vi "Create RPC Method.vi"(8 "error in (no error)":errorcluster, 10 "RPC Method Parameters":T1, 11 "Server class in":refnum<vi>) -> (0 "error out":errorcluster, 2 "Newly created ?":bool, 3 "Server class out":refnum<vi>)   [LabVIEW 2019, in "gRPC Scripting Tools.lvlib"]
uses:
  gRPC Scripting Tools.lvlib
  TypeDefs/RPC Method Parameters.ctl
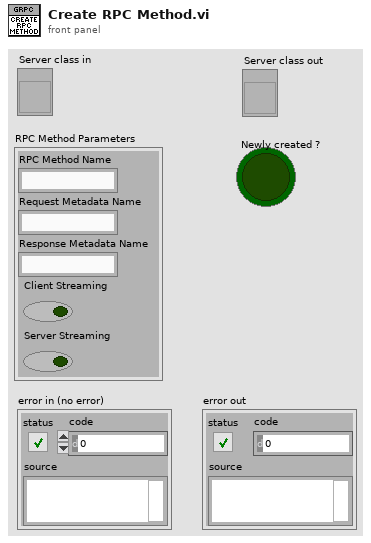
[diagram p1: front panel]
types:
  T1 = typedef "gRPC Scripting Tools.lvlib/RPC Method Parameters.ctl" = cluster{"RPC Method Name":string, "Request Metadata Name":string, "Response Metadata Name":string, "Client Streaming":bool, "Server Streaming":bool}
  T2 = enum32{"invalid VI type", "Standard VI", "Control VI", "Global VI", "Polymorphic VI", "Configuration VI", "SubSystem", "Facade VI", "Method VI"}
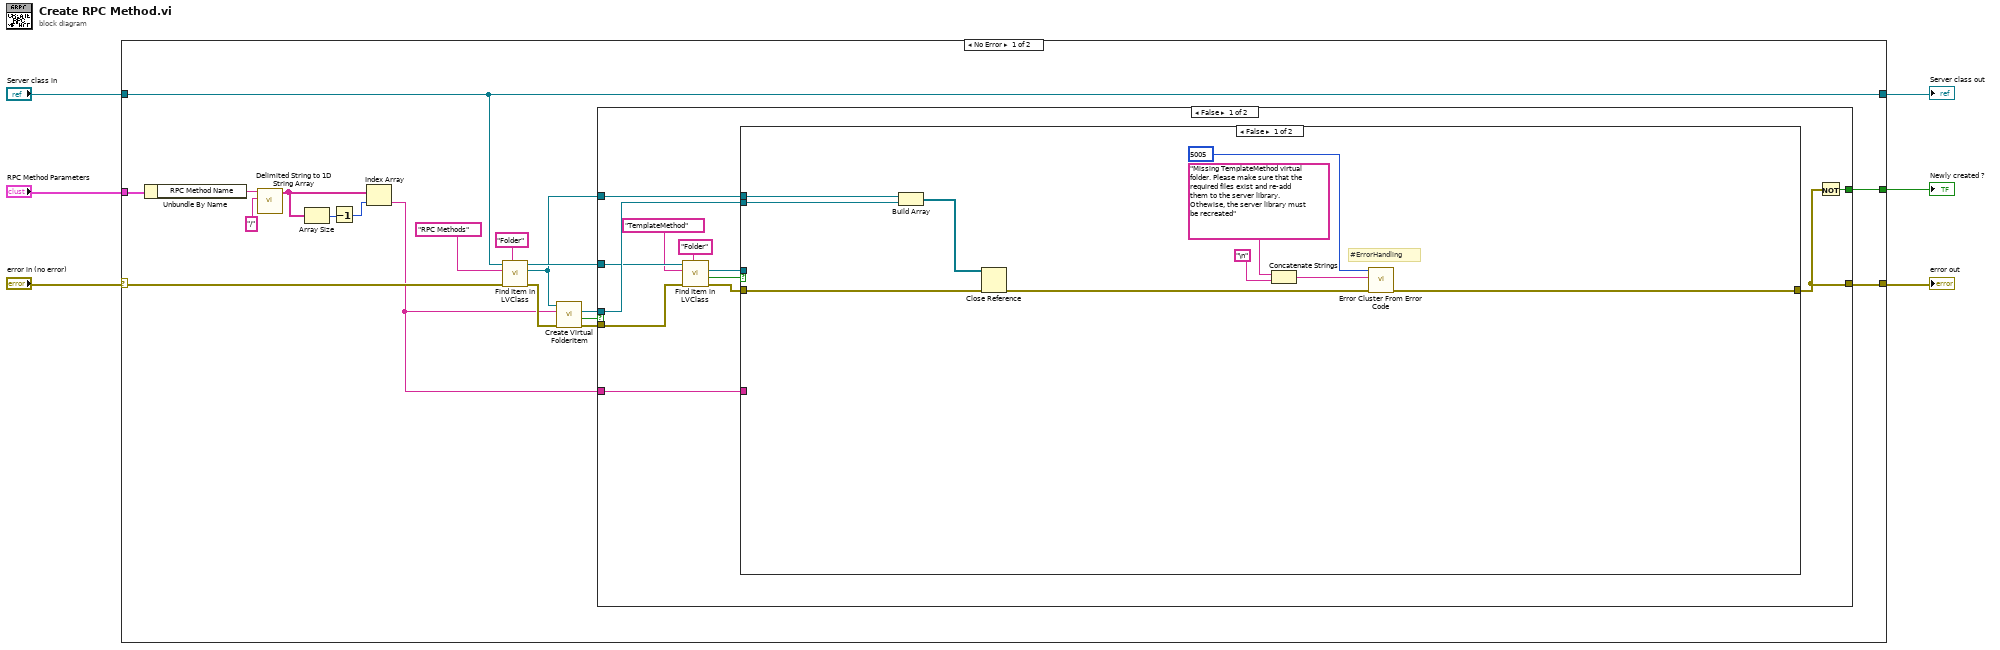
[diagram p0: block diagram]
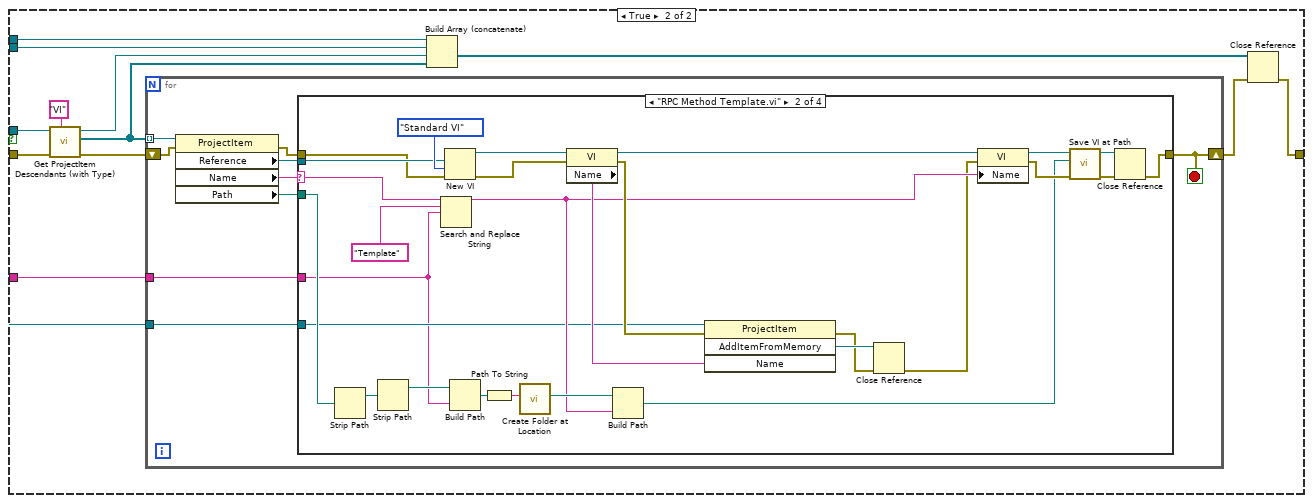
[diagram p2: hidden frame]
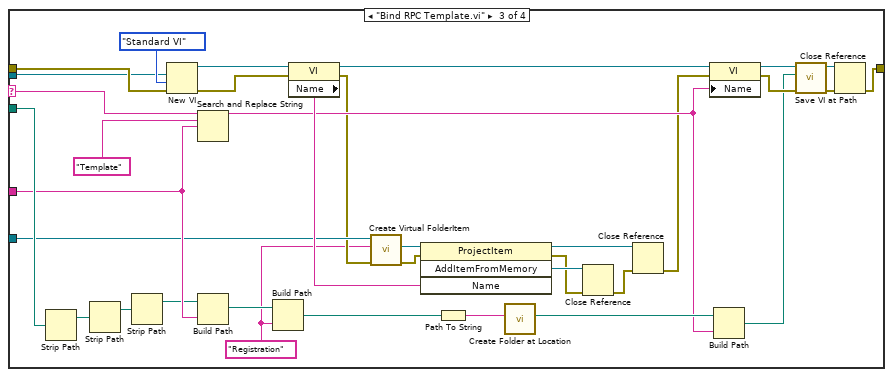
[diagram p4: hidden frame]
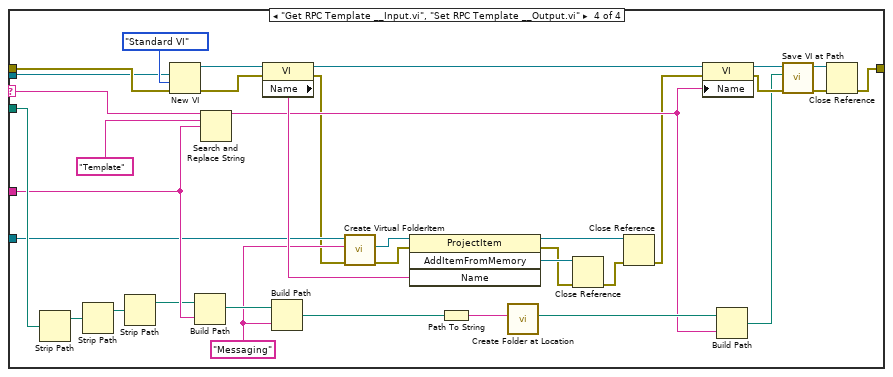
[diagram p5: hidden frame]
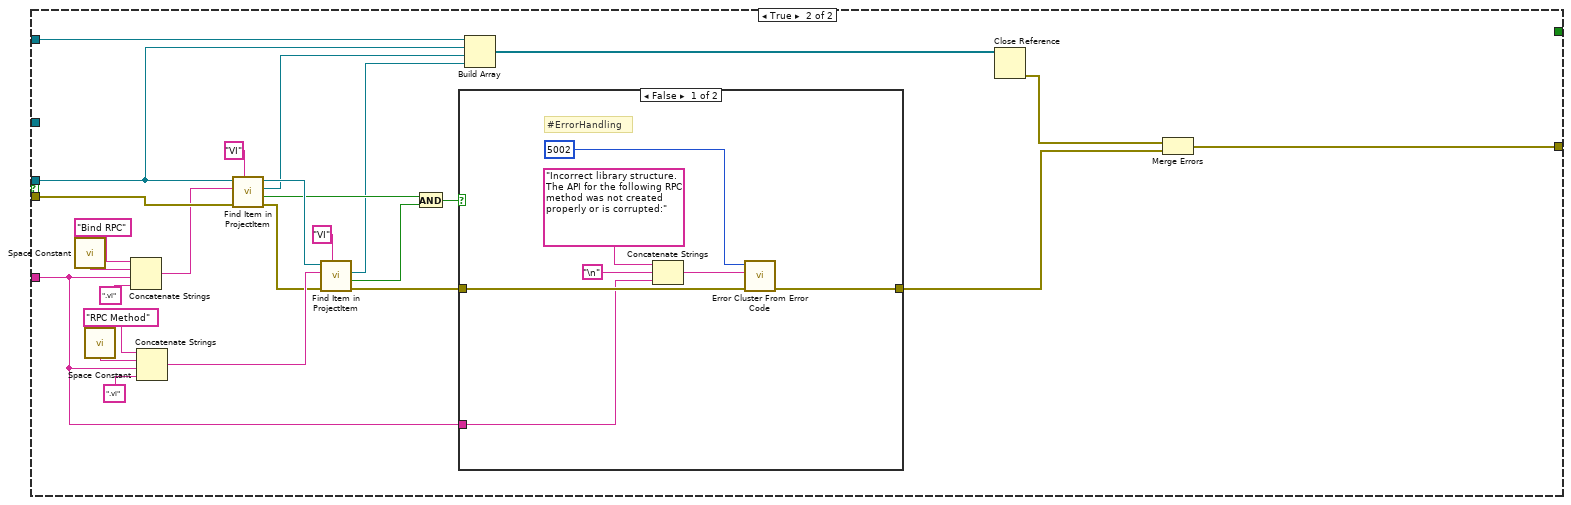
[diagram p6: hidden frame]
diagram:
  n1 = case shown="No Error" "error in (no error)" {
    selector: "error in (no error)" -> [w16 w203]
    tunnel: "Server class in" -> [w15 w202]
    tunnel: [w21 w203] -> w5
    tunnel: [w15 w202] -> w3
    tunnel: [w14 _] -> w2
    tunnel: "RPC Method Parameters" -> [w7 _]
    frame No Error {
      n2 = Unbundle By Name(w7) -> ("RPC Method Name"=w10:string)
      n3 = call <vilib>:"Delimited String to 1D String Array.vi"("delimiter"="/", "delimited string"=w10) -> ("string array"=w13:string[])  [unwired: 9 in]
      n4 = Array Size(array=w13) -> (size(s)=w11:i32)
      n5 = Decrement(x=w11) -> (x-1=w12:i32)
      n6 = Index Array(array=w13, index=w12) -> (element=w8:string)
      n7 = call "Find Item in LVClass.vi"("Item Type"="Folder", "error in (no error)"=w16, "Item Name"="RPC Methods", "Class Item in"=w15) -> ("error out"=w20:errorcluster, "Project Item (Class Item)"=w18:refnum<vi>, "Class Item out"=w22:refnum<vi>)  [unwired: 4 in, 1 out]
      n8 = call "Create Virtual FolderItem.vi"("error in (no error)"=w20, "Folder Name"=w8, "ProjectItem in"=w18) -> ("error out"=w19:errorcluster, "Already exists?"=w25:bool, "FolderItem reference out"=w17:refnum<vi>)  [unwired: 5 in, 1 out]
      n9 = case shown="False" w25 {
        tunnel: w17 -> [w37 w176]
        tunnel: w18 -> [w36 w177]
        tunnel: w19 -> [w35 w192]
        tunnel: [w30 w168] -> w21
        tunnel: w22 -> [w34 _]
        tunnel: w8 -> [w31 w172]
        tunnel: [w29 _] -> w14
        frame False {
          n10 = call "Find Item in LVClass.vi"("Item Type"="Folder", "error in (no error)"=w35, "Item Name"="TemplateMethod", "Class Item in"=w34) -> ("error out"=w27:errorcluster, "Found?"=w26:bool, "Project Item (Class Item)"=w28:refnum<vi>)  [unwired: 4 in, 1 out]
          n11 = case shown="False" w26 {
            tunnel: w37 -> [w41 w59]
            tunnel: w36 -> [w42 w58]
            tunnel: w31 -> [_ w56]
            tunnel: [w43 w55] -> w30
            tunnel: w28 -> [_ w54]
            tunnel: w27 -> [w40 w53]
            frame False {
              # "#ErrorHandling"
              n12 = Build Array(w42, w41) -> (w39:refnum<vi>[])
              n13 = Close Reference(reference=w39, error in (no error)=w40) -> (error out=w38:errorcluster)
              n14 = Concatenate Strings("Missing TemplateMethod virtual folder. Please make sure that the required files exist and re-add them to the server library. Othewise, the server library must be recreated" ("error message (\"\")"), "\n") -> (w44:string)
              n15 = call <vilib>:"Error Cluster From Error Code.vi"("error in (no error)"=w38, "error message (\"\")"=w44, "error code (0)"=5005) -> ("error out"=w43:errorcluster)  [unwired: 6 in]
            }
            frame True {
              n16 = call "Get ProjectItem Descendants (with Type).vi"("Type"="VI", "error in (no error)"=w53, "ProjectItem in"=w54) -> ("error out"=w49:errorcluster, "All Descendents"=w50:refnum<vi>[], "ProjectItem out"=w51:refnum<vi>)  [unwired: 6 in]
              n17 = for {
                tunnel: w50 -> [w68] mode=indexing
                tunnel: w59 -> [w62]
                tunnel: w56 -> [w63]
                shift-right: [w60] -> w48
                shift-left: w49 -> [w67]
                stop <- w60 stop-if-true
                n18 = property class="ProjectItem"(reference=w68, error in=w67) -> (error out=w61:errorcluster, "Reference"=w65:refnum<vi>, "Name"=w66:string, "Path"=w64:path)  [unwired: 1 out]
                n19 = case shown="\"RPC Method Template.vi\"" w66 {
                  selector: w66 -> [_ w75 w113 w146]
                  tunnel: w65 -> [_ w76 w114 w147]
                  tunnel: w64 -> [_ w74 w112 w145]
                  tunnel: w63 -> [_ w70 w111 w144]
                  tunnel: w62 -> [_ w73 w105 w140]
                  tunnel: w61 -> [w69 w72 w115 w148]
                  tunnel: [w69 w71 w108 w143] -> w60
                  frame "None", Default {
                  }
                  frame "RPC Method Template.vi" {
                    n20 = Strip Path(path=w74) -> (stripped path=w77:path)  [unwired: 1 out]
                    n21 = Strip Path(path=w77) -> (stripped path=w88:path)  [unwired: 1 out]
                    n22 = Search and Replace String(input string=w75, search string="Template", replace string=w70) -> (result string=w84:string)  [unwired: 5 in, 3 out]
                    n23 = New VI(8:w72, 9:T2."Standard VI" ("vi type (standard vi)"), 10:w76) -> (0:w92:errorcluster, 3:w95:refnum<vi>)  [unwired: 1 in, 3 out]
                    n24 = Build Path(base path=w88, name or relative path=w70) -> (appended path=w87:path)
                    n25 = Path To String(path=w87) -> (string=w86:string)
                    n26 = call "Create Folder at Location.vi"("Path"=w86) -> ("Full path out"=w85:path)  [unwired: 8 in, 2 out]
                    n27 = property class="VI"(reference=w95, error in=w92) -> (reference out=w93:refnum<vi>, error out=w91:errorcluster, "Name"=w96:string)
                    n28 = Build Path(base path=w85, name or relative path=w84) -> (appended path=w83:path)
                    n29 = invoke class="ProjectItem" method="AddItemFromMemory"(reference=w73, error in=w91, "Name"=w96) -> (error out=w79:errorcluster, "AddItemFromMemory"=w80:refnum<vi>)  [unwired: 1 in, 2 out]
                    n30 = Close Reference(reference=w80, error in (no error)=w79) -> (error out=w78:errorcluster)
                    n31 = property class="VI"(reference=w93, error in=w78, "Name"=w84) -> (reference out=w90:refnum<vi>, error out=w89:errorcluster)
                    n32 = call "Save VI at Path.vi"("error in (no error)"=w89, "Path"=w83, "VI in"=w90) -> ("error out"=w82:errorcluster, "VI out"=w81:refnum<vi>)  [unwired: 6 in, 1 out]
                    n33 = Close Reference(reference=w81, error in (no error)=w82) -> (error out=w71:errorcluster)
                  }
                  frame "Bind RPC Template.vi" {
                    w103 = "Registration" ("name or relative path")
                    n34 = Strip Path(path=w112) -> (stripped path=w116:path)  [unwired: 1 out]
                    n35 = Strip Path(path=w116) -> (stripped path=w107:path)  [unwired: 1 out]
                    n36 = Strip Path(path=w107) -> (stripped path=w106:path)  [unwired: 1 out]
                    n37 = New VI(8:w115, 9:T2."Standard VI" ("vi type (standard vi)"), 10:w114) -> (0:w127:errorcluster, 3:w130:refnum<vi>)  [unwired: 1 in, 3 out]
                    n38 = Search and Replace String(input string=w113, search string="Template", replace string=w111) -> (result string=w122:string)  [unwired: 5 in, 3 out]
                    n39 = Build Path(base path=w106, name or relative path=w111) -> (appended path=w110:path)
                    n40 = Build Path(base path=w110, name or relative path=w103) -> (appended path=w109:path)
                    n41 = property class="VI"(reference=w130, error in=w127) -> (reference out=w128:refnum<vi>, error out=w104:errorcluster, "Name"=w131:string)
                    n42 = call "Create Virtual FolderItem.vi"("error in (no error)"=w104, "Folder Name"=w103, "ProjectItem in"=w105) -> ("error out"=w101:errorcluster, "FolderItem reference out"=w102:refnum<vi>)  [unwired: 5 in, 2 out]
                    n43 = invoke class="ProjectItem" method="AddItemFromMemory"(reference=w102, error in=w101, "Name"=w131) -> (reference out=w100:refnum<vi>, error out=w117:errorcluster, "AddItemFromMemory"=w118:refnum<vi>)  [unwired: 1 in, 1 out]
                    n44 = Path To String(path=w109) -> (string=w124:string)
                    n45 = call "Create Folder at Location.vi"("Path"=w124) -> ("Full path out"=w123:path)  [unwired: 8 in, 2 out]
                    n46 = Close Reference(reference=w118, error in (no error)=w117) -> (error out=w99:errorcluster)
                    n47 = Close Reference(reference=w100, error in (no error)=w99) -> (error out=w98:errorcluster)
                    n48 = property class="VI"(reference=w128, error in=w98, "Name"=w122) -> (reference out=w126:refnum<vi>, error out=w125:errorcluster)
                    n49 = Build Path(base path=w123, name or relative path=w122) -> (appended path=w121:path)
                    n50 = call "Save VI at Path.vi"("error in (no error)"=w125, "Path"=w121, "VI in"=w126) -> ("error out"=w120:errorcluster, "VI out"=w119:refnum<vi>)  [unwired: 6 in, 1 out]
                    n51 = Close Reference(reference=w119, error in (no error)=w120) -> (error out=w108:errorcluster)
                  }
                  frame "Get RPC Template __Input.vi", "Set RPC Template __Output.vi" {
                    w137 = "Messaging" ("name or relative path")
                    n52 = Strip Path(path=w145) -> (stripped path=w151:path)  [unwired: 1 out]
                    n53 = Strip Path(path=w151) -> (stripped path=w142:path)  [unwired: 1 out]
                    n54 = Strip Path(path=w142) -> (stripped path=w141:path)  [unwired: 1 out]
                    n55 = New VI(8:w148, 9:T2."Standard VI" ("vi type (standard vi)"), 10:w147) -> (0:w162:errorcluster, 3:w165:refnum<vi>)  [unwired: 1 in, 3 out]
                    n56 = Build Path(base path=w141, name or relative path=w144) -> (appended path=w150:path)
                    n57 = Search and Replace String(input string=w146, search string="Template", replace string=w144) -> (result string=w157:string)  [unwired: 5 in, 3 out]
                    n58 = property class="VI"(reference=w165, error in=w162) -> (reference out=w163:refnum<vi>, error out=w136:errorcluster, "Name"=w166:string)
                    n59 = Build Path(base path=w150, name or relative path=w137) -> (appended path=w149:path)
                    n60 = call "Create Virtual FolderItem.vi"("error in (no error)"=w136, "Folder Name"=w137, "ProjectItem in"=w140) -> ("error out"=w138:errorcluster, "FolderItem reference out"=w139:refnum<vi>)  [unwired: 5 in, 2 out]
                    n61 = invoke class="ProjectItem" method="AddItemFromMemory"(reference=w139, error in=w138, "Name"=w166) -> (reference out=w135:refnum<vi>, error out=w152:errorcluster, "AddItemFromMemory"=w153:refnum<vi>)  [unwired: 1 in, 1 out]
                    n62 = Path To String(path=w149) -> (string=w159:string)
                    n63 = call "Create Folder at Location.vi"("Path"=w159) -> ("Full path out"=w158:path)  [unwired: 8 in, 2 out]
                    n64 = Close Reference(reference=w153, error in (no error)=w152) -> (error out=w134:errorcluster)
                    n65 = Close Reference(reference=w135, error in (no error)=w134) -> (error out=w133:errorcluster)
                    n66 = property class="VI"(reference=w163, error in=w133, "Name"=w157) -> (reference out=w161:refnum<vi>, error out=w160:errorcluster)
                    n67 = Build Path(base path=w158, name or relative path=w157) -> (appended path=w156:path)
                    n68 = call "Save VI at Path.vi"("error in (no error)"=w160, "Path"=w156, "VI in"=w161) -> ("error out"=w155:errorcluster, "VI out"=w154:refnum<vi>)  [unwired: 6 in, 1 out]
                    n69 = Close Reference(reference=w154, error in (no error)=w155) -> (error out=w143:errorcluster)
                  }
                }
              }
              n70 = Build Array (concatenate)(w58, w59, w51, w50) -> (w57:refnum<vi>[])
              n71 = Close Reference(reference=w57, error in (no error)=w48) -> (error out=w55:errorcluster)
            }
          }
          n72 = Not(x=w30) -> (.not. x?=w29:bool)
        }
        frame True {
          n73 = call <vilib>:"Space Constant.vi"() -> ("String"=w185:string)
          n74 = call <vilib>:"Space Constant.vi"() -> ("String"=w184:string)
          n75 = Concatenate Strings("Bind RPC" ("string"), w185, w172, ".vi" ("string")) -> (w188:string)
          n76 = Concatenate Strings("RPC Method" ("string"), w184, w172, ".vi" ("string")) -> (w182:string)
          n77 = call "Find Item in ProjectItem.vi"("Item Type"="VI" ("Type"), "error in (no error)"=w192, "Name"=w188, "ProjectItem in"=w176) -> ("error out"=w181:errorcluster, "Found ?"=w180:bool, "Item Refnum out"=w175:refnum<vi>, "ProjectItem out"=w190:refnum<vi>)  [unwired: 4 in]
          n78 = call "Find Item in ProjectItem.vi"("Item Type"="VI" ("Type"), "error in (no error)"=w181, "Name"=w182, "ProjectItem in"=w190) -> ("error out"=w173:errorcluster, "Found ?"=w179:bool, "Item Refnum out"=w174:refnum<vi>)  [unwired: 4 in, 1 out]
          n79 = And(x=w180, y=w179) -> (x .and. y?=w178:bool)
          n80 = case shown="False" w178 {
            tunnel: w173 -> [w200 w201]
            tunnel: w172 -> [w196 _]
            tunnel: [w194 w201] -> w170
            frame False {
              # "#ErrorHandling"
              n81 = Concatenate Strings("Incorrect library structure. The API for the following RPC method was not created properly or is corrupted:" ("error message (\"\")"), "\n", w196) -> (w195:string)
              n82 = call <vilib>:"Error Cluster From Error Code.vi"("error in (no error)"=w200, "error message (\"\")"=w195, "error code (0)"=5002) -> ("error out"=w194:errorcluster)  [unwired: 6 in]
            }
            frame True {
            }
          }
          n83 = Build Array(w177, w176, w175, w174) -> (w171:refnum<vi>[])
          n84 = Close Reference(reference=w171) -> (error out=w169:errorcluster)  [unwired: 1 in]
          n85 = Merge Errors(w169, w170) -> (w168:errorcluster)
        }
      }
    }
    frame Error {
    }
  }
  "error out" <- w5
  "Server class out" <- w3
  "Newly created ?" <- w2
